vi "create restart FPGA command.vi"() -> (3 "command message":variant)   [LabVIEW 2018, in "RT - FPGA commands.lvlib"]
uses:
  RT - FPGA commands.lvlib
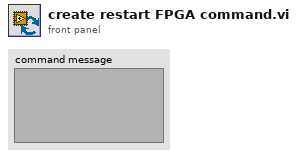
[diagram p1: front panel]
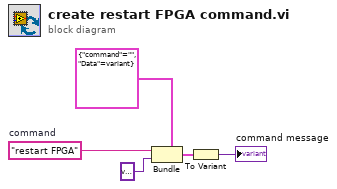
[diagram p0: block diagram]
diagram:
  w4 = "restart FPGA"  # command
  n1 = Bundle(cluster=cluster{"command":string, "Data":variant} {"command"="", "Data"=variant}, "command"=w4, "Data"=variant) -> (w3:cluster{"command":string, "Data":variant})
  n2 = To Variant(anything=w3) -> (Variant=→"command message":variant)
